vi "START_STOP_SEND.vi"(8 "error in (no error)":errorcluster, 10 "START/STOP":bool, 11 "CONTADOR_CON_LIMITES in":refnum<class "CONTADOR_CON_LIMITES.lvclass">) -> (0 "error out":errorcluster, 3 "CONTADOR_CON_LIMITES out":refnum<class "CONTADOR_CON_LIMITES.lvclass">)   [LabVIEW 2019, in "CONTADOR_CON_LIMITES.lvlib" / "CONTADOR_CON_LIMITES.lvclass"]
uses:
  CONTADOR_CON_LIMITES.lvclass
  CONTADOR_CON_LIMITES.lvclass/CONTADOR_CON_LIMITES.ctl
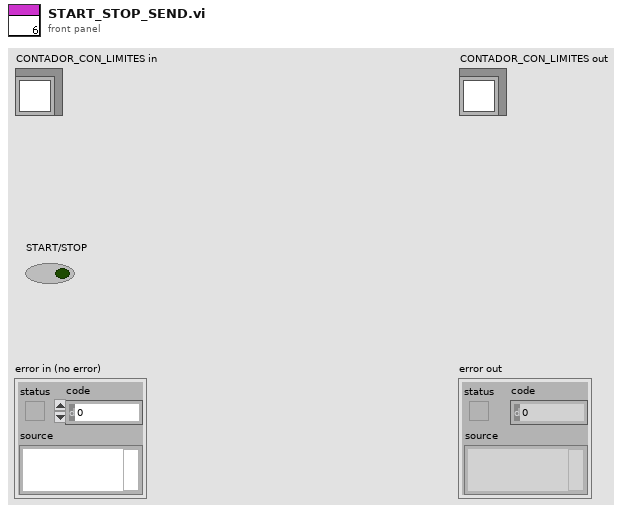
[diagram p1: front panel]
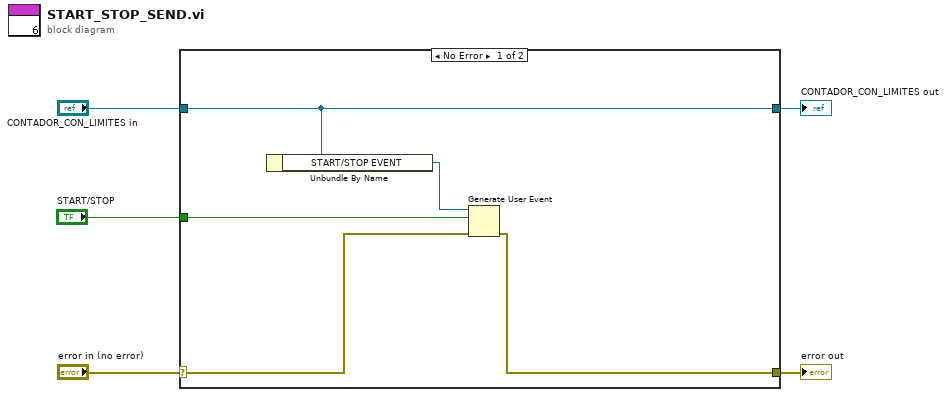
[diagram p0: block diagram]
diagram:
  n1 = case shown="No Error" "error in (no error)" {
    selector: "error in (no error)" -> [w7 w12]
    tunnel: [w6 w12] -> w4
    tunnel: [w10 w11] -> w2
    tunnel: "CONTADOR_CON_LIMITES in" -> [w10 w11]
    tunnel: "START/STOP" -> [w8 _]
    frame No Error {
      n2 = Unbundle By Name(w10) -> ("START/STOP EVENT"=w9:refnum<user-event>)
      n3 = Generate User Event(user event=w9, event data cluster=w8, error in=w7) -> (error out=w6:errorcluster)  [unwired: 1 in, 1 out]
    }
    frame Error {
    }
  }
  "error out" <- w4
  "CONTADOR_CON_LIMITES out" <- w2
